vi "Create.vi"(8 "error in (no error)":errorcluster) -> (0 "error out":errorcluster, 3 "Result Model out":refnum<class "Result Model by Reference.lvclass">)   [LabVIEW 2020, in "Result Model by Reference.lvclass"]
uses:
  Result Model by Reference.lvclass
  Result Model/Result Model.lvclass
  Core/Result/Result.ctl
  Core/Result/Status.ctl
  Core/Result/Type.ctl
  Result Model by Reference.lvclass/Result Model by Reference.ctl
  Core/Result/Result.lvlib
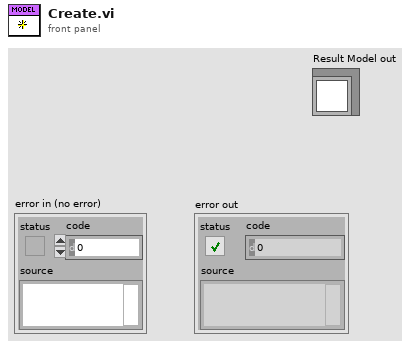
[diagram p1: front panel]
types:
  T1 = typedef "Result.lvlib/Result.ctl" = cluster{"Name":string, "Description":string, "Status":T2, "Result Type":T3, "Execution Time":dbl, "Data":cluster{"Expected":variant, "Actual":variant, "Delta":variant}}
  T2 = typedef "Result.lvlib/Status.ctl" = enum16{"", "Passed", "Failed", "Error", "Skipped", "Setup Error", "Broken", "Teardown Error"}
  T3 = typedef "Result.lvlib/Type.ctl" = enum16{"Test Case", "Test Suite", "Test Run", "Pass", "Fail", "Skip", "Pass if", "Fail if", "Pass if Error", "Fail if Error", "Pass if Equal", "Fail if Equal"}
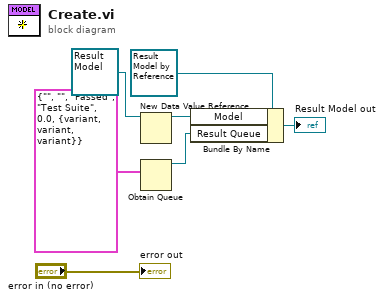
[diagram p0: block diagram]
diagram:
  n1 = New Data Value Reference(data value=refnum<class "Result Model.lvclass"> refnum ("Result Model.lvclass")) -> (data value reference=w3:refnum<data-value>)  [unwired: 1 in, 1 out]
  n2 = Obtain Queue(element data type=T1 {"Name"="", "Description"="", "Status"=enum."Passed", "Result Type"=enum."Test Suite", "Execution Time"=0.0, "Data"={"Expected"=variant, "Actual"=variant, "Delta"=variant}} ("Results")) -> (queue out=w1:refnum<queue>)  [unwired: 4 in, 2 out]
  n3 = Bundle By Name(cluster=refnum<class "Result Model by Reference.lvclass"> refnum ("Result Model in"), "Model"=w3, "Result Queue"=w1) -> (→"Result Model out":refnum<class "Result Model by Reference.lvclass">)
  "error out" <- "error in (no error)"
